vi "ROI grp-window ini.vi"() -> (0 "error out":errorcluster, 3 "ROI groups new setup":T1 {"Groups setup out"."Group region specifier cluster"."Contours"."Type" items=["No Selection", "Point", "Line", "Rectangle", "Oval", "Polygon", "Freehand Region", "Annulus", "Unused2", "Unused3", "Broken Line", "Freehand Line", "Rotated Rectangle"]})   [LabVIEW 2020]
uses:
  Typedefs/ROI grp-Internal register.ctl
  ROI Selection Interface/ROI group info cluster.ctl
  Typedefs/Group sel cluster.ctl
  Experiment header interface/Typedefs/Save-Load-Save as-Load last enum.ctl
  Typedefs/Get-Set-Clear Control.ctl
  Globals/gl_ROI grp window globals.vi
  Global variables/gl_Functional Imaging-Global variables.vi
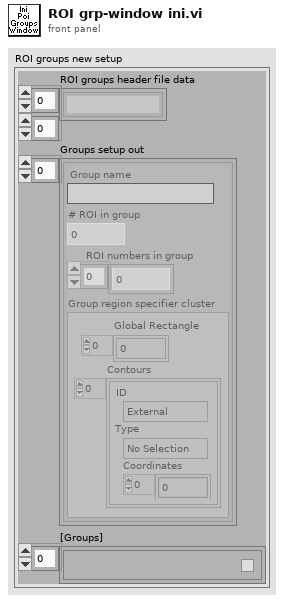
[diagram p1: front panel]
types:
  T1 = typedef "ROI grp-Internal register.ctl" = cluster{"ROI groups header file data":string[][], "Groups setup out":T2[], "[Groups]":T4[]}
  T2 = typedef "ROI group info cluster.ctl" = cluster{"Group name":string, "# ROI in group":i32, "ROI numbers in group":i32[], "Group region specifier cluster":T3}
  T3 = typedef "ROI Descriptor" = cluster{"Global Rectangle":i32[], "Contours":cluster{"ID":enum32{"External", "Internal"}, "Type":u32, "Coordinates":i32[]}[]}
  T4 = typedef "Group sel cluster.ctl" = cluster{"Group number":string, "Group Name":string, "Visibility":bool, "Highlight":bool}
  T5 = typedef "Get-Set-Clear Control.ctl" = enum16{"Get", "Set", "Clear"}
  T6 = typedef "Save-Load-Save as-Load last enum.ctl" = enum16{"Save file", "Save file as", "Load file", "Load last file"}
  T7 = typedef "Functional Imging UI Refs.ctl" = cluster{"Menu ref":refnum<k9>, "Image control":refnum<vi>, "VI ref":refnum<vi>, "XGrapher":refnum<vi>, "Smoothing":refnum<vi>, "POI Averaging":refnum<vi>, "Normalize":refnum<vi>, "POI data points in each trial":refnum<vi>, "Channel":refnum<vi>, "Experiment data folder path":refnum<vi>, "[ROI vis]":refnum<vi>, "[Groups] visbl":T8, "Group Name":refnum<vi>, "POI index":refnum<vi>, "Trial No.":refnum<vi>, "Intensity Zoom":refnum<vi>, "Trial Cursor Enabled":refnum<vi>, "Number of Trials (ind 1)":refnum<vi>, "Number of Trials (ind 2)":refnum<vi>, "MiniScans Available":refnum<vi>, "POI Available":refnum<vi>, "Defer graph updates":refnum<vi>, "Waveform selector":refnum<vi>, "#of selected POI":refnum<vi>, "#of selected MiniScans":refnum<vi>, "#of selected groups":refnum<vi>, "Max Z-Projection":refnum<vi>, "Z-Plane Selector":refnum<vi>, "Index of miniscan point to visualise":refnum<vi>, "ROI vis. mode":refnum<vi>, "Total # of points":refnum<vi>, "Index of group clicked on":refnum<vi>, "Pane 1":refnum<vi>, "Pane 2":refnum<vi>, "Pane 3":refnum<vi>, "Pane 4":refnum<vi>, "Pane 5":refnum<vi>, "Pane 6":refnum<vi>, "Deselect all ROI":refnum<vi>, "Deselect all groups":refnum<vi>}
  T8 = typedef "Groups array referecne.ctl" = refnum<vi>
  T9 = typedef "ROI grp-window ctrl refs.ctl" = cluster{"This VI":refnum<vi>, "Pane":refnum<vi>, "Table":refnum<vi>}
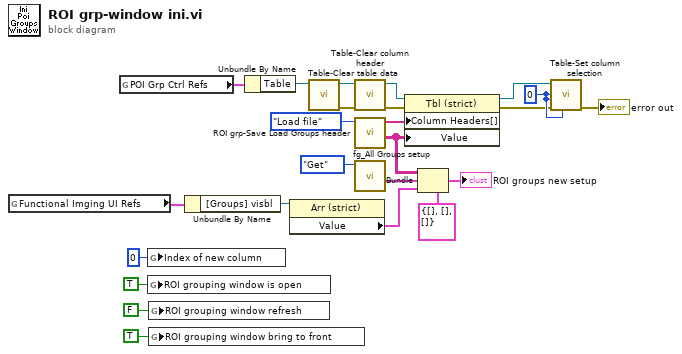
[diagram p0: block diagram]
diagram:
  w21 = 0 ("Index of row to select")
  n1 = global read "gl_Functional Imaging-Global variables.vi" "Functional Imging UI Refs"() -> (w4:T7)
  n2 = global read "gl_ROI grp window globals.vi" "POI Grp Ctrl Refs"() -> (w13:T9)
  n3 = global write "gl_ROI grp window globals.vi" "Index of new column"(0 ("Index of new column")) -> ()
  n4 = global write "gl_ROI grp window globals.vi" "ROI grouping window is open"(TRUE ("Groups vis window is open")) -> ()
  n5 = global write "gl_ROI grp window globals.vi" "ROI grouping window refresh"(FALSE ("Groups vis window refresh")) -> ()
  n6 = global write "gl_ROI grp window globals.vi" "ROI grouping window bring to front"(TRUE ("Bring POI grouping window to front")) -> ()
  n7 = Unbundle By Name(w4) -> ("[Groups] visbl"=w3:T8)
  n8 = Unbundle By Name(w13) -> ("Table"=w24:refnum<vi>)
  n9 = property on="Property Node" class="Arr (strict)"(reference=w3) -> ("Value"=w2:T4[])  [unwired: 1 in, 2 out]
  n10 = call <userlib>:"Table-Clear table data.vi"("Table in"=w24) -> ("error out"=w23:errorcluster, "Table out"=w22:refnum<vi>)  [unwired: 9 in]
  n11 = call <userlib>:"Table-Clear column header.vi"("error in (no error)"=w23, "Table in"=w22) -> ("error out"=w18:errorcluster, "Table out"=w17:refnum<vi>)  [unwired: 8 in]
  n12 = call "ROI grp-Save Load Groups header.vi"("Function"=Save-Load-Save_as-Load_last_enum."Load file") -> ("POI groups header file data"=w5:string[][], "POI groups column header"=w16:string[])  [unwired: 8 in, 1 out]
  n13 = call "fg_All Groups setup.vi"("Function"=Get-Set-Clear_Control."Get") -> ("Groups setup out"=w8:T2[])  [unwired: 9 in, 1 out]
  n14 = property on="Property Node" class="Tbl (strict)"(reference=w17, error in=w18, "Column Headers[]"=w16, "Value"=w5) -> (reference out=w20:refnum<vi>, error out=w19:errorcluster)
  n15 = Bundle(cluster=T1 {"ROI groups header file data"=[], "Groups setup out"=[], "[Groups]"=[]} ("ROI groups new setup"), "ROI groups header file data"=w5, "Groups setup out"=w8, "[Groups]"=w2) -> (→"ROI groups new setup":T1)
  n16 = call <userlib>:"Table-Set column selection.vi"("Selection length (i.e. Number of rows)"=w21, "error in (no error)"=w19, "Index of column to select"=w21, "Index of row to select"=w21, "Table in"=w20) -> ("error out"=→"error out":errorcluster)  [unwired: 5 in, 1 out]
